vi "排序.vi"(1 "排序前":string[][](array[string])) -> (0 "排序后":string[][](array[string]))   [LabVIEW 2019]
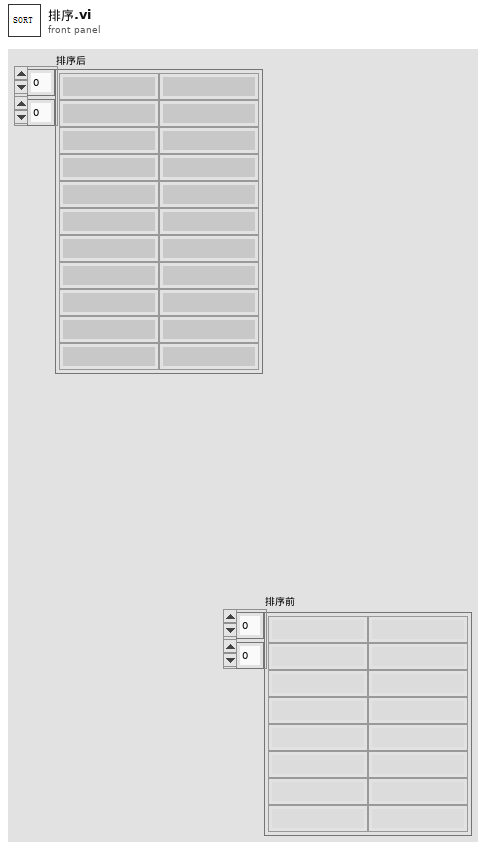
[diagram p1: front panel]
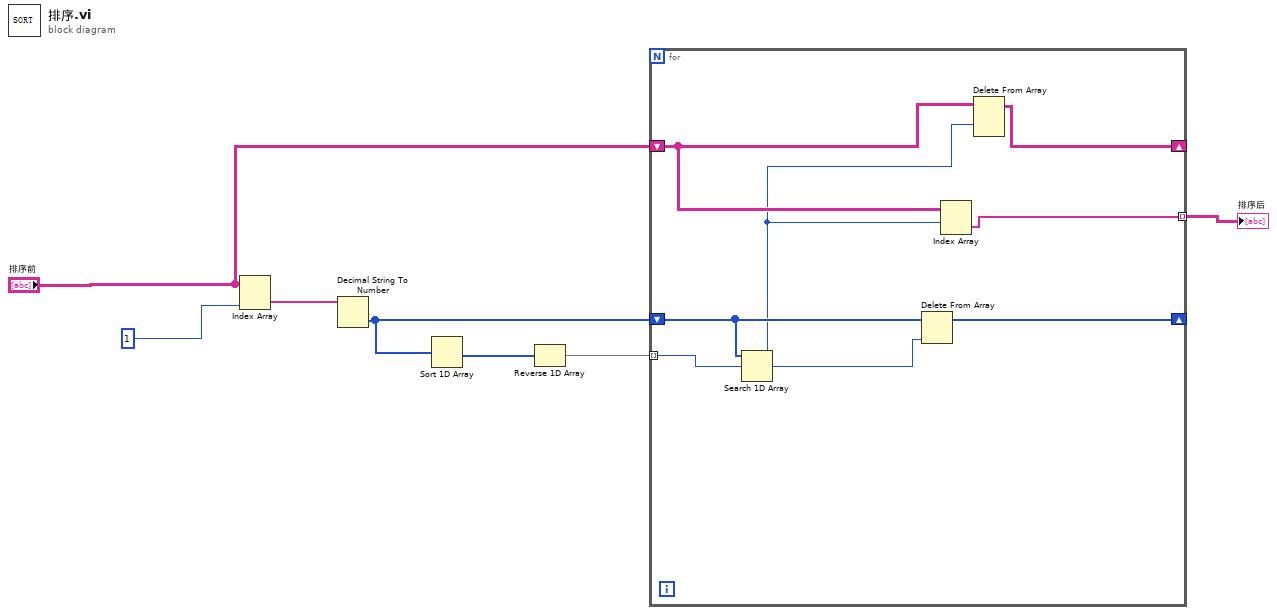
[diagram p0: block diagram]
diagram:
  n1 = Index Array(array="排序前", index (col)=1 ("索引")) -> (element=w6:string[])  [unwired: 1 in]
  n2 = Decimal String To Number(string=w6) -> (number=w3:i32[])  [unwired: 2 in, 1 out]
  n3 = Sort 1D Array(array=w3) -> (sorted array=w5:i32[])
  n4 = Reverse 1D Array(array=w5) -> (reversed array=w4:i32[])
  n5 = for {
    tunnel: w4 -> [w14] mode=indexing
    shift-right: [w9] -> _
    shift-left: "排序前" -> [w11]
    shift-right: [w12] -> _
    shift-left: w3 -> [w13]
    tunnel: [w8] -> w2 mode=indexing
    n6 = Search 1D Array(1D array=w13, element=w14) -> (index of element=w10:i32)  [unwired: 1 in]
    n7 = Delete From Array(array=w13, index=w10) -> (array with subset deleted=w12:i32[])  [unwired: 1 in, 1 out]
    n8 = Index Array(array=w11, index (row)=w10) -> (element=w8:string[])  [unwired: 1 in]
    n9 = Delete From Array(array=w11, index (row)=w10) -> (array with subset deleted=w9:string[][])  [unwired: 2 in, 1 out]
  }
  "排序后" <- w2
